vi "导出波形.vi"(0 "WaveTime":dbl[](array[numeric]), 1 "WaveData":dbl[][](array[numeric]), 3 "错误输入":errorcluster, 4 "保存路径":path) -> (5 "列数":i32, 8 "错误输出":errorcluster)   [LabVIEW 2018]
uses:
  <vilib>/Utility/file.llb/Write Delimited Spreadsheet (string).vi
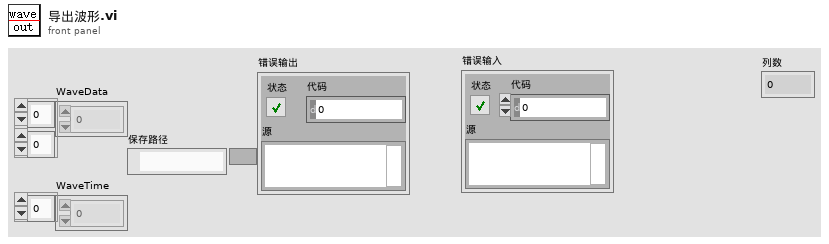
[diagram p1: front panel]
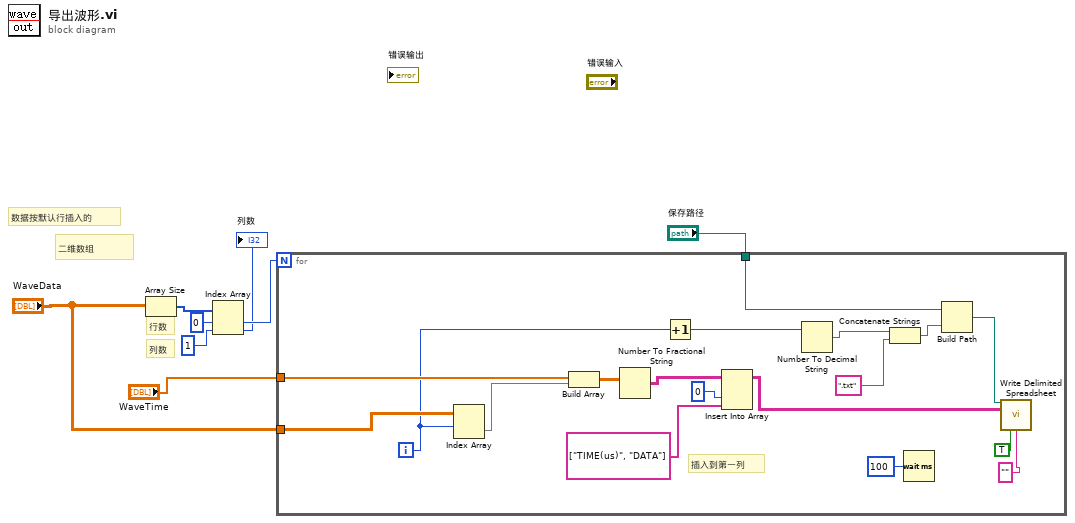
[diagram p0: block diagram]
diagram:
  # "二维数组"
  # "数据按默认行插入的"
  # "列数"
  # "行数"
  n1 = Array Size(array="WaveData") -> (size(s)=w8:i32[])
  n2 = Index Array(array=w8, index #1=0 ("索引"), index #2=1 ("索引")) -> (element #1=w6:i32, element #2=→"列数":i32)
  n3 = for {
    N: w6 -> [_]
    tunnel: "WaveData" -> [w16]
    tunnel: "WaveTime" -> [w14]
    tunnel: "保存路径" -> [w13]
    i -> [w11]
    # "插入到第一列"
    n4 = Index Array(array=w16, index (row)=w11) -> (element=w15:dbl[])  [unwired: 1 in]
    n5 = Build Array(w14, w15) -> (w26:dbl[][])
    n6 = Number To Fractional String(number=w26) -> (F-format string=w25:string[][])  [unwired: 3 in]
    n7 = Increment(x=w11) -> (x+1=w10:i32)
    n8 = Insert Into Array(array=w25, index (col)=0 ("禁用的索引 (列)"), new element=string[] ["TIME(us)", "DATA"]) -> (w9:string[][])  [unwired: 1 in]
    n9 = Number To Decimal String(number=w10) -> (decimal integer string=w19:string)  [unwired: 1 in]
    n10 = Concatenate Strings(w19, ".txt" ("名称或相对路径")) -> (w18:string)
    n11 = Wait (ms)(milliseconds to wait=u32 100 ("等待时间（毫秒）")) -> ()  [unwired: 1 out]
    n12 = Build Path(base path=w13, name or relative path=w18) -> (appended path=w21:path)
    n13 = call-poly <vilib>:"Write Delimited Spreadsheet.vi"("file path (dialog if empty)"=w21, "2D data"=w9, "transpose? (no:F)"=TRUE, "delimiter (\\t)"="" ("delimiter (\\t)")) -> ()  [unwired: 10 in, 2 out]
  }
